vi "FileGen_Update status ind.vi"(11 "Cluster":T1={"Imaging Protocol"=enum."Live Imaging", "Number of Trials"=0, "Frame Size"=512, "# Averaged frames"=0, "Dwell time (us)"=0.0, "Index of Z-plane"=0, "Timelapse?"=FALSE, "Logging process is active"=FALSE, "Speed logging enabled"=FALSE, "tdms file ref"=refnum, "path"=path "", "Trial Number"=0, "Expected # points acquired"=FALSE, "Manually stopped"=FALSE, "Last trial"=FALSE, "Ch0 data"=[], "Ch1 data"=[], "Ref Data"=[], "Ref Frame Time"=[], "Image Time"=[], "Continuous Time"=[], "Ref X Length"=0, "Ref Y Length"=0, "# Ref Averaged frames"=0, "Ref Dwell time (us)"=0.0, "Points acquired"={"Ch0 last trial"=0, "Ch1 last trial"=0, "All trials"=0}, "HW Timings File"=refnum} {"Ref Dwell time (us)" format="%#.6g"; "Frame Size" items=["100X100"=100, "128X128"=128, "200X200"=200, "256X256"=256, "512X512"=512, "1024x1024"=1024, "2048x2048"=2048]; "Dwell time (us)" format="%#.6g"}) -> (0 "error out":errorcluster)   [LabVIEW 2020]
uses:
  Typedefs/Logging queue element.ctl
  Typedefs/Imaging Protocols enum.ctl
  Typedefs/Frame Size.ctl
  Typedefs/Acquired points count.ctl
  Global Variables/gl_Queues.vi
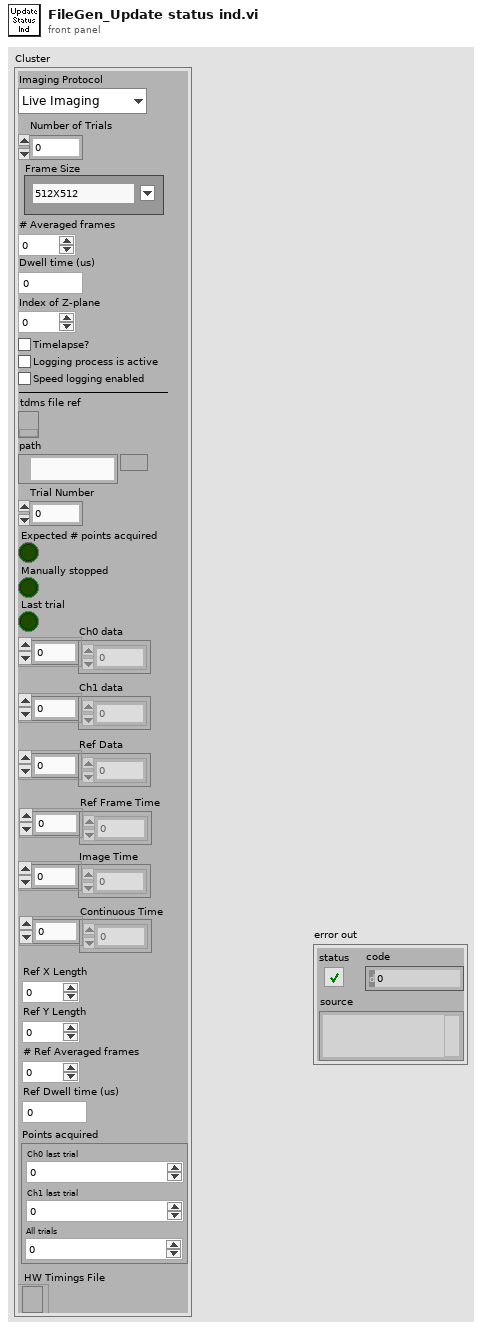
[diagram p1: front panel]
types:
  T1 = typedef "Logging queue element.ctl" = cluster{"Imaging Protocol":T2, "Number of Trials":u16, "Frame Size":T3, "# Averaged frames":u16, "Dwell time (us)":dbl, "Index of Z-plane":i32, "Timelapse?":bool, "Logging process is active":bool, "Speed logging enabled":bool, "tdms file ref":refnum<k34>, "path":path, "Trial Number":i32, "Expected # points acquired":bool, "Manually stopped":bool, "Last trial":bool, "Ch0 data":u32[], "Ch1 data":u32[], "Ref Data":u32[], "Ref Frame Time":u64[], "Image Time":u64[], "Continuous Time":u64[], "Ref X Length":u16, "Ref Y Length":u16, "# Ref Averaged frames":u16, "Ref Dwell time (us)":dbl, "Points acquired":T4, "HW Timings File":refnum<file>}
  T2 = typedef "Imaging Protocols enum.ctl" = enum16{"AOL Z-Stack", "Motor Z Stack", "Functional Acquisition", "Single Plane Acquisition", "Volume Acquisition", "Live Imaging", "Live Plane Imaging", "Live Volume Imaging"}
  T3 = typedef "Frame Size.ctl" = u16
  T4 = typedef "Acquired points count.ctl" = cluster{"Ch0 last trial":u64, "Ch1 last trial":u64, "All trials":u64}
  T5 = typedef "All Message Queues.ctl" = cluster{"UI queue":refnum<queue>, "Acq. queue":refnum<queue>, "Logging queue":refnum<queue>}
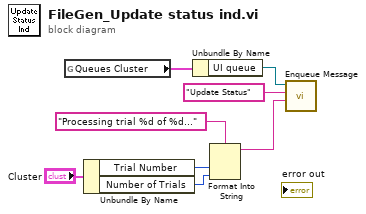
[diagram p0: block diagram]
diagram:
  n1 = global read "gl_Queues.vi" "Queues Cluster"() -> (w1:T5)
  n2 = Unbundle By Name("Cluster") -> ("Trial Number"=w3:i32, "Number of Trials"=w2:u16)
  n3 = Unbundle By Name(w1) -> ("UI queue"=w6:refnum<queue>)
  n4 = Format Into String(format string="Processing trial %d of %d..." ("Acquiring and Logging..."), w3, w2) -> (resulting string=w4:string)  [unwired: 2 in, 1 out]
  n5 = call "Enqueue Message.vi"("Message Data"=w4, "Message"="Update Status", "Queue"=w6) -> ()  [unwired: 7 in, 2 out]
